vi "XNET Reflective Memory Initialization VI.vi"(8 "error in (no error)":errorcluster, 10 "Custom XML":string, 11 "Device Item Ref in":T1 format="%.0x") -> (0 "error out":errorcluster, 3 "Device Item Ref out":T1 format="%.0x")   [LabVIEW 2010, in "XNET Reflective Memory Custom Device.lvlib"]
uses:
  XNET Reflective Memory Custom Device.lvlib
  <vilib>/NI VeriStand/Custom Device API/Custom Device Item Ref.ctl
  <vilib>/NI Veristand/Custom Device API/Custom Device API.lvlib
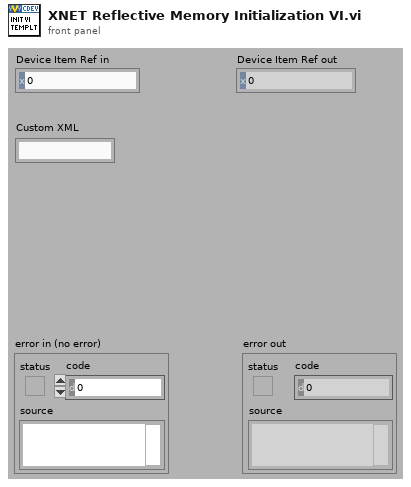
[diagram p1: front panel]
types:
  T1 = typedef "Custom Device API.lvlib/Custom Device Item Ref.ctl" = u64
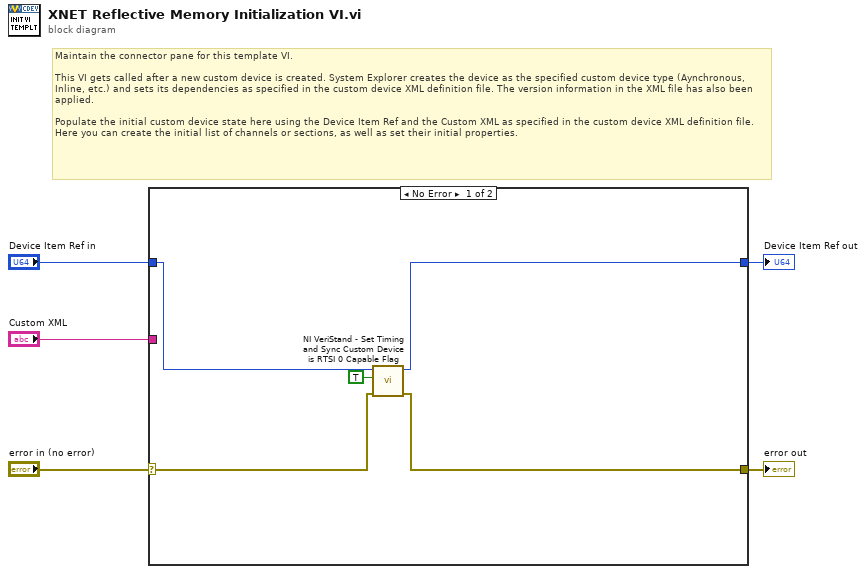
[diagram p0: block diagram]
diagram:
  # "Maintain the connector pane for this template VI.\n\nThis VI gets called after a new custom device is created. System Explorer creates the device as the specified custom device type (Aynchronous, Inline, etc.) and sets its dependencies as specified in the custom device XML definition file. The version information in the XML file has also been applied.\n\nPopulate the initial custom device state here using the Device Item Ref and the Custom XML as specified in the custom device XML definition file. Here you can create the initial list of channels or sections, as well as set their initial properties."
  n1 = case shown="No Error" "error in (no error)" {
    selector: "error in (no error)" -> [w10 w12]
    tunnel: [w9 w12] -> w5
    tunnel: [w7 w11] -> w3
    tunnel: "Device Item Ref in" -> [w8 w11]
    tunnel: "Custom XML" -> [_ _]
    frame No Error {
      n2 = call <vilib>:"NI VeriStand - Set Timing and Sync Custom Device is RTSI 0 Capable Flag.vi"("error in (no error)"=w10, "Is RTSI 0 Capable"=TRUE, "Device Ref in"=w8) -> ("error out"=w9:errorcluster, "Device Ref out"=w7:T1)  [unwired: 7 in]
    }
    frame Error {
    }
  }
  "error out" <- w5
  "Device Item Ref out" <- w3
